vi "Autonomous Independent.vi"   [LabVIEW 2017]
doc: "This VI is called when autonomous begins, and will automatically be terminated when autonomous ends. You can carry out timed or sensor driven robot movement independently without needing to return to the caller."
uses:
  TypeDef/ENUM_Drive_ACT Loop_Mode.ctl
  <vilib>/Rock Robotics/Network Tables/NT Read String.vi
  Systems/WC_Drive/Global_SM Write_Data Out.vi
  Systems/Joystick/Global_Joystick Write_Data.vi
  Systems/WC_Drive/Global_WC_Drive_Zero_Encoders.vi
  Systems/Joystick/Joystick.lvlib
panel:
  # "Be sure to right-click and choose Data Operations>>Make Current Value default if you want to save the array values with the VI"
types:
  T1 = typedef "ENUM_Drive_ACT Loop_Mode.ctl" = enum16{"Stop", "Position", "VBus", "Profile"}
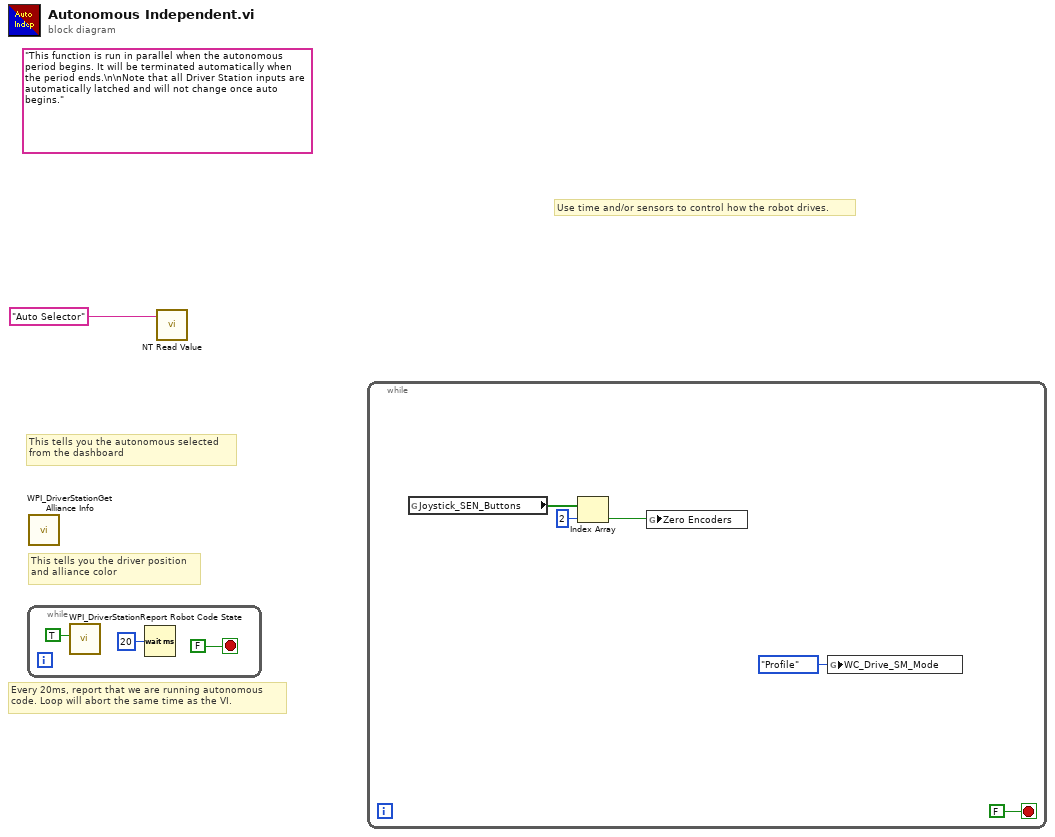
[diagram p0: block diagram]
diagram:
  (unwired) "This function is run in parallel when the autonomous period begins. It will be terminated automatically when the period ends.\n\nNote that all Driver Station inputs are automatically latched and will not change once auto begins."
  # "This tells you the autonomous selected\nfrom the dashboard"
  # "Every 20ms, report that we are running autonomous\ncode. Loop will abort the same time as the VI."
  # "Use time and/or sensors to control how the robot drives."
  # "This tells you the driver position\nand alliance color"
  n1 = while {
    stop <- FALSE stop-if-true
    n2 = call <vilib>:"WPI_DriverStationReport Robot Code State.vi"("Autonomous"=TRUE) -> ()  [unwired: 10 in, 1 out]
    n3 = Wait (ms)(milliseconds to wait=u32 20) -> ()  [unwired: 1 out]
  }
  n4 = call <vilib>:"WPI_DriverStationGet Alliance Info.vi"() -> ()  [unwired: 12 out]
  n5 = call-poly <vilib>:"NT Read Value.vi"("Name"="Auto Selector") -> ()  [unwired: 9 in, 2 out]
  n6 = while {
    stop <- FALSE stop-if-true
    n7 = global read "Global_Joystick Write_Data.vi" "Joystick_SEN_Buttons"() -> (w7:bool[])
    n8 = Index Array(array=w7, index=2) -> (element=w5:bool)
    n9 = global write "Global_WC_Drive_Zero_Encoders.vi" "Zero Encoders"(w5) -> ()
    n10 = global write "Global_SM Write_Data Out.vi" "WC_Drive_SM_Mode"(ENUM_Drive_ACT_Loop_Mode."Profile" ("WC_Drive_SM_Mode")) -> ()
  }
